vi "Main Editor UI.vi"() -> ()   [LabVIEW 2015, in "Increment editor node.lvclass"]
doc: "This is the main view for configuration the behavior of a module in the DCAF standard editor."
uses:
  Increment editor node.lvclass
  <vilib>/NI/Configuration Framework/Node/NodeRef.ctl
  <vilib>/NI/Configuration Framework/Node/NISE_CEF_Node.lvclass
  <vilib>/NI/AMC/Message Queue.ctl
  <vilib>/NI/AMC/Message.ctl
  <vilib>/NI/Tools/Keyed Array/KeyedArray.ctl
  <vilib>/NI/Configuration Framework/Node/UserEventRef.ctl
  <vilib>/NI/Configuration Framework/Controls/EventCluster.ctl
  <vilib>/NI/DCAF UI Toolkit/Controls/Configure.ctl
  <vilib>/NI/DCAF UI Toolkit/Controls/Add.ctl
  <vilib>/NI/DCAF UI Toolkit/Controls/Remove.ctl
  <vilib>/NI/Configuration Framework/Node/StopEvent.ctl
  <vilib>/NI/Configuration Framework/Node/RefreshUIEvent.ctl
  <vilib>/NI/Configuration Framework/Node/CacheState.ctl
  <vilib>/NI/Configuration Framework/Node/NodeChangeEvent.ctl
  <vilib>/NI/Tag Bus/tag/Data Type.ctl
  Permissions Enum.ctl
  <vilib>/NI/DCAF/Tag Editor Core/Table API/Available Tag Menu/channel action event.ctl
  <vilib>/NI/DCAF/Tag Editor Core/Table API/Available Tag Menu/dialog output action.ctl
  <vilib>/NI/Tag Bus Module Framework/channel/TBM channel.lvclass
  <vilib>/NI/Tag Bus/tag/tag descriptor.lvclass
  <vilib>/NI/DCAF/Tag Editor Core/Table API/Table Manager/Call Back Ref Type Def.ctl
  <vilib>/NI/DCAF/Tag Editor Core/Configuration Editor/Classes/Engine Parent/Engine Parent Editor Node.lvclass
  <vilib>/NI/DCAF/Tag Editor Core/Configuration Editor/Classes/Module editor node/module editor node.lvclass
  <vilib>/NI/DCAF UI Toolkit/Controls/Import.ctl
  <vilib>/NI/DCAF UI Toolkit/Controls/Export.ctl
  <vilib>/NI/DCAF/Tag Editor Core/Table API/Table Manager/references.ctl
  <vilib>/Utility/miscctls.llb/LVPositionTypeDef.ctl
  <vilib>/NI/DCAF/Tag Editor Core/Table API/Listbox/Multi Column Listbox.lvclass
  <vilib>/NI/Configuration Framework/NISE_CEF_TreeControl.lvlib
  <vilib>/NI/Tools/Keyed Array/Tools_KeyedArray.lvlib
  <vilib>/NI/AMC/AMC.lvlib
  <vilib>/NI/DCAF/Tag Editor Core/Table API/Table Manager.lvlib
  <vilib>/NI/DCAF/Tag Editor Core/Table API/Table Manager/Table Manager.lvclass
  <vilib>/NI/DCAF UI Toolkit/Controls/DCAF UI Elements.lvlib
panel:
  in  "user event out":refnum<user-event>
  in  "Permissions":T1
  in  "data type":T2
  in  "node change":T3
  in  "cache state":T4
  in  "refresh UI":T5
  in  "stop event":T6
  in  "Tab Control":enum32{"Channel Configuration", "Import Export"}(tab)
  in  "Remove Button":T7
  in  "Add Button":T8
  in  "Table":i32(listbox)
  in  "settings":T9
  in  "Export":T10
  in  "Import":T11
  in  "user event":T12
  in  "main queue":T13
  in  "node ref":T14
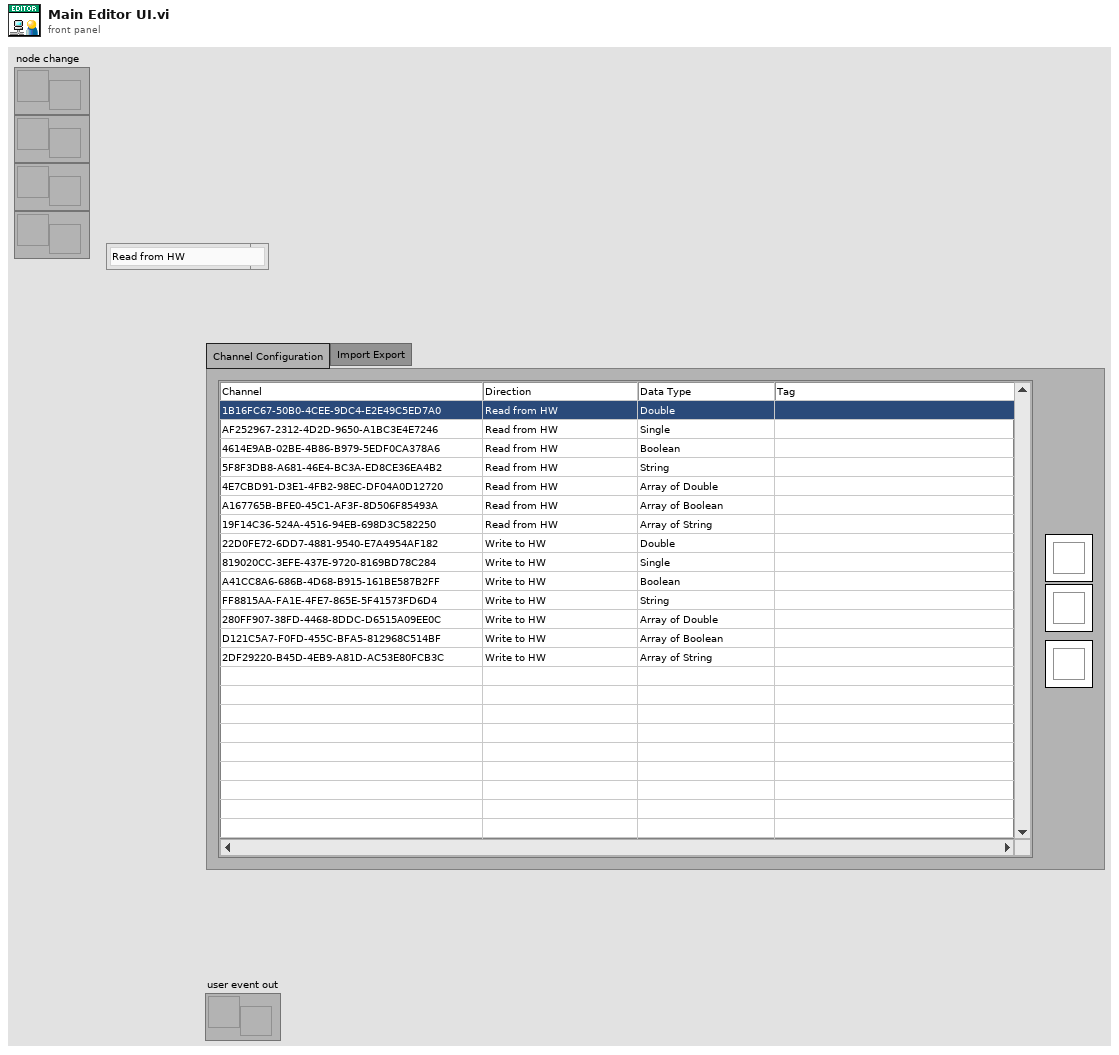
[diagram p1: front panel]
types:
  T1 = typedef "Increment editor node.lvclass/Permissions Enum.ctl" = enum16{"Read from HW", "Write to HW"}
  T2 = typedef "tag bus.lvlib/tag descriptor.lvclass/Data Type.ctl" = enum16{"Double", "Single", "I64", "I32", "I16", "I8", "U64", "U32", "U16", "U8", "Boolean", "String", "Array of Double", "Array of Single", "Array of I64", "Array of I32", "Array of I16", "Array of I8", "Array of U64", "Array of U32", "Array of U16", "Array of U8", "Array of Boolean", "Array of String"}
  T3 = typedef "NISE_CEF_Node.lvclass/NodeChangeEvent.ctl" = refnum<user-event>
  T4 = typedef "NISE_CEF_Node.lvclass/CacheState.ctl" = refnum<user-event>
  T5 = typedef "NISE_CEF_Node.lvclass/RefreshUIEvent.ctl" = refnum<user-event>
  T6 = typedef "NISE_CEF_Node.lvclass/StopEvent.ctl" = refnum<user-event>
  T7 = typedef "DCAF UI Elements.lvlib/Remove.ctl" = bool
  T8 = typedef "DCAF UI Elements.lvlib/Add.ctl" = bool
  T9 = typedef "DCAF UI Elements.lvlib/Configure.ctl" = bool
  T10 = typedef "DCAF UI Elements.lvlib/Export.ctl" = bool
  T11 = typedef "DCAF UI Elements.lvlib/Import.ctl" = bool
  T12 = typedef "NISE_CEF_Node.lvclass/UserEventRef.ctl" = refnum<user-event>
  T13 = typedef "AMC.lvlib/Message Queue.ctl" = refnum<queue>
  T14 = typedef "NISE_CEF_Node.lvclass/NodeRef.ctl" = refnum<data-value>
  T15 = typedef "Table Manager.lvlib/Table Manager.lvclass/references.ctl" = cluster{"stop event":T6, "refresh UI":T5, "cache state":T4, "node change":T3, "user event out":refnum<user-event>, "main queue":T13, "user event":T12}
  T16 = typedef "LVPositionTypeDef.ctl" = cluster{"Left":i32, "Top":i32}
  T17 = typedef "Table Manager.lvlib/Table Manager.lvclass/object ref.ctl" = cluster{"engine":refnum<data-value>, "Node Ref":refnum<data-value>}
  T18 = typedef "Table Manager.lvlib/Column.lvclass/Column Descriptor.ctl" = cluster{"name":string, "caption":string, "Column Type":T19, "Params":string, "AutoSizeMode":i32, "FillWeight":sgl, "MinWidth":u32, "tooltip":string, "Enum Reference":refnum<vi>, "Channel suffix":string, "Read Only":bool, "Call Back VI":T20, "DT Dependency":i32, "name dependency":i32, "data type":T2, "Custom Column":refnum<class "Column.lvclass">}
  T19 = typedef "Table Manager.lvlib/Column.lvclass/Column Type.ctl" = enum16{"String", "Mapping", "Enum", "Custom"}
  T20 = typedef "Table Manager.lvlib/Table Manager.lvclass/Call Back Ref Type Def.ctl" = refnum<vi>
  T21 = typedef "Table Manager.lvlib/Table Manager.lvclass/Table Events.ctl" = cluster{"Menu Selection":refnum<user-event>}
  T22 = enum8{"Enabled", "Disabled", "Disabled and Grayed Out"}
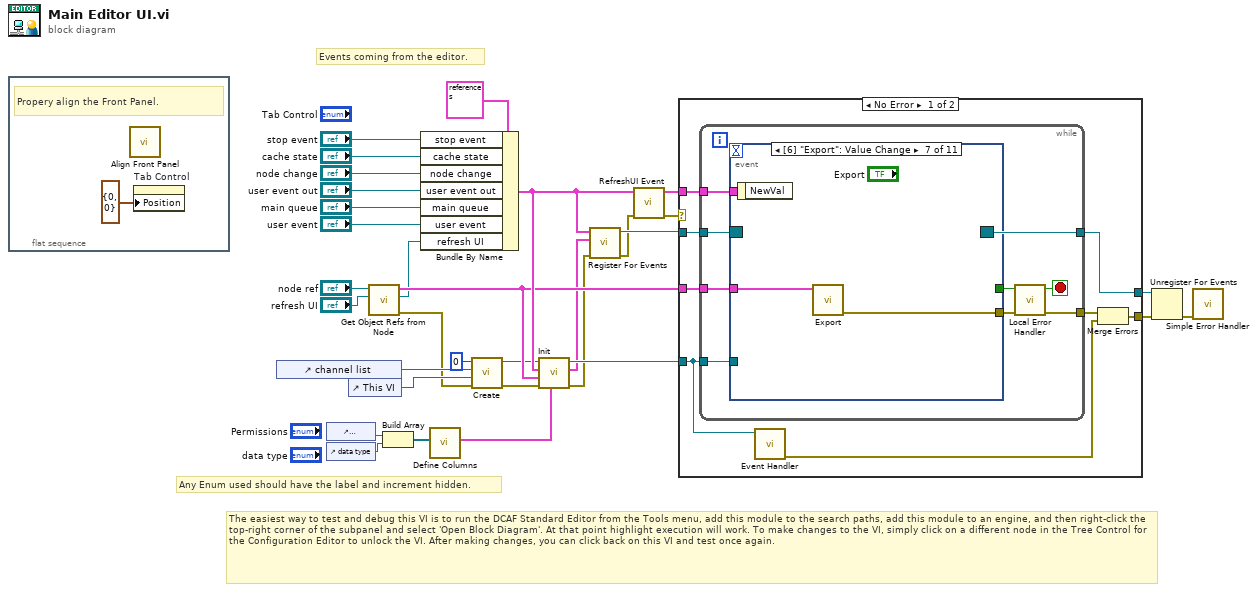
[diagram p0: block diagram]
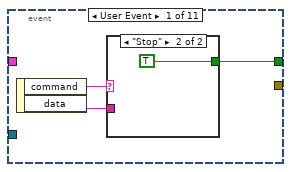
[diagram p2: hidden frame]
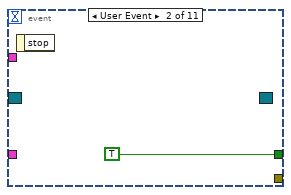
[diagram p4: hidden frame]
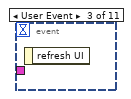
[diagram p5: hidden frame]
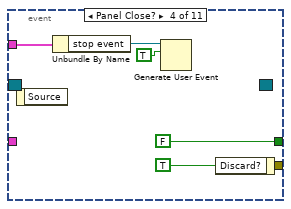
[diagram p6: hidden frame]
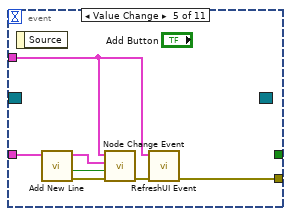
[diagram p7: hidden frame]
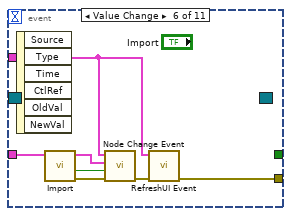
[diagram p8: hidden frame]
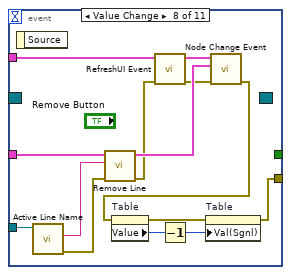
[diagram p9: hidden frame]
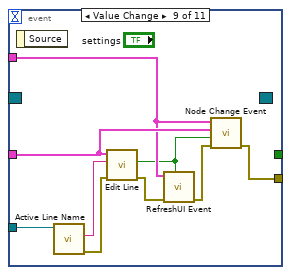
[diagram p10: hidden frame]
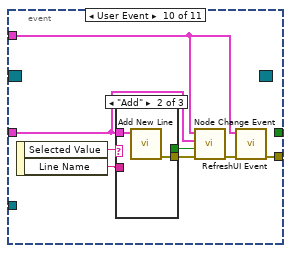
[diagram p11: hidden frame]
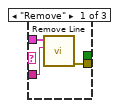
[diagram p12: hidden frame]
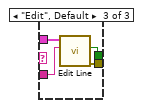
[diagram p13: hidden frame]
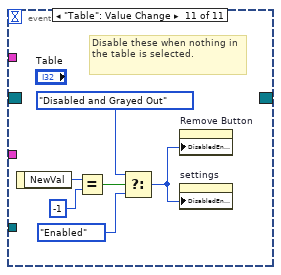
[diagram p14: hidden frame]
diagram:
  # "The easiest way to test and debug this VI is to run the DCAF Standard Editor from the Tools menu, add this module to the search paths, add this module to an engine, and then right-click the top-right corner of the subpanel and select 'Open Block Diagram'. At that point highlight execution will work. To make changes to the VI, simply click on a different node in the Tree Control for the Configuration Editor to unlock the VI. After making changes, you can click back on this VI and test once again."
  # "Any Enum used should have the label and increment hidden."
  # "Events coming from the editor."
  n1 = flat-sequence {
    frame #0 {
      # "Propery align the Front Panel."
      n2 = call <vilib>:"Align Front Panel.vi"() -> ()  [unwired: 10 in, 2 out]
      n3 = property on="Tab Control" class="TabCtl (strict)"("Position"=T16 {"Left"=0, "Top"=0}) -> ()  [unwired: 2 in, 2 out]
    }
  }
  n4 = control-ref of="channel list"() -> (w8:refnum<vi>)
  n5 = control-ref of="Permissions"() -> (w18:refnum<vi>)
  n6 = control-ref of="data type"() -> (w17:refnum<vi>)
  n7 = control-ref of="This VI"() -> (w6:refnum<vi>)
  n8 = call "Get Object Refs from Node.vi"("Refresh UI"="refresh UI", "Data Value Reference in"="node ref") -> ("error out"=w3:errorcluster, "Refresh UI out"=w1:T5, "References"=w15:T17)  [unwired: 7 in]
  n9 = Build Array(w18, w17) -> (w16:refnum<vi>[])
  n10 = Bundle By Name(cluster=T15 {"stop event"=refnum, "refresh UI"=refnum, "cache state"=refnum, "node change"=refnum, "user event out"=refnum, "main queue"=refnum, "user event"=refnum} ("References"), "stop event"="stop event", "cache state"="cache state", "node change"="node change", "user event out"="user event out", "main queue"="main queue", "user event"="user event", "refresh UI"=w1) -> (w19:T15)
  n11 = call "Define Columns.vi"("Enum Array"=w16) -> ("Column Definition"=w21:T18[])  [unwired: 10 in]
  n12 = call <vilib>:"Create.vi"("error in (no error)"=w3, "Top VI"=w6, "Listbox"=w8, "Index"=0) -> ("error out"=w4:errorcluster, "reference out"=w5:refnum<class "Multi Column Listbox.lvclass">)  [unwired: 6 in]
  n13 = call-dynamic "Init.vi"("Column Descriptors"=w21, "error in (no error)"=w4, "Node object refs"=w15, "Event References"=w19, "Multi Column Listbox in"=w5) -> ("error out"=w10:errorcluster, "Table Events"=w9:T21, "Multi Column Listbox out"=w14:refnum<class "Multi Column Listbox.lvclass">)  [unwired: 4 in]
  n14 = call "Register For Events.vi"("error in"=w10, "Table Events"=w9, "References"=w19) -> ("error out"=w12:errorcluster, "Event Registration Refnum"=w22:refnum<event-registration>)  [unwired: 7 in]
  n15 = call "RefreshUI Event.vi"("error in (no error)"=w12, "References in"=w19) -> ("error out"=w11:errorcluster, "References out"=w20:T15)  [unwired: 8 in]
  n16 = case shown="No Error" w11 {
    selector: w11 -> [_ w122]
    tunnel: w22 -> [w41 w121]
    tunnel: [w40 w121] -> w32
    tunnel: [w34 w122] -> w31
    tunnel: w20 -> [w39 _]
    tunnel: w15 -> [w38 _]
    tunnel: w14 -> [w37 _]
    frame No Error {
      n17 = while {
        tunnel: w41 -> [w50]
        tunnel: [w49] -> w40
        tunnel: [w46] -> w35
        tunnel: w39 -> [w44]
        tunnel: w38 -> [w43]
        tunnel: w37 -> [w42]
        stop <- w48 stop-if-true
        n18 = event shown="[6] \"Export\": Value Change" {
          selector: w50 -> [_ _ _ _ _ _ _ _ _ _ _]
          dyn-events: [_ _ _ _ _ _ _ _ _ _ _] -> w49
          timeout: _ -> [_ _ _ _ _ _ _ _ _ _ _]
          tunnel: [w53 TRUE _ FALSE _ _ _ _ _ _ _] -> w47
          tunnel: [_ _ _ _ w61 w71 w74 w77 w97 w103 _] -> w45
          tunnel: w44 -> [_ _ _ w57 w65 w73 _ w88 w92 w99 _]
          tunnel: w43 -> [_ _ _ _ w66 w70 w75 w87 w95 w100 _]
          tunnel: w42 -> [_ _ _ _ _ _ _ w83 w96 _ _]
          event User Event {
            n19 = event-data() -> ("command"=w52:string, "data"=w51:string)  [unwired: 1 in]
            n20 = case shown="\"Stop\"" w52 {
              tunnel: [_ TRUE] -> w53
              tunnel: w51 -> [_ _]
              frame Default {
              }
              frame "Stop" {
              }
            }
          }
          event User Event {
            n21 = event-data() -> ()  [unwired: 1 in, 1 out]
          }
          event User Event {
            n22 = event-data() -> ()  [unwired: 1 in, 1 out]
          }
          event Panel Close? {
            n23 = event-data() -> ()  [unwired: 1 in, 1 out]
            n24 = Unbundle By Name(w57) -> ("stop event"=w56:T6)
            n25 = Generate User Event(user event=w56, event data cluster=TRUE ("event data")) -> ()  [unwired: 2 in, 2 out]
            n26 = event-data("Discard?"=TRUE) -> ()  [unwired: 1 in, 1 out]
          }
          event Value Change {
            n27 = event-data() -> ()  [unwired: 1 in, 1 out]
            n28 = call "Add New Line.vi"("objects"=w66) -> ("error out"=w64:errorcluster, "success"=w62:bool)  [unwired: 8 in, 1 out]
            n29 = call "Node Change Event.vi"("error in (no error)"=w64, "Send (T)"=w62, "objects"=w66, "References in"=w65) -> ("error out"=w63:errorcluster)  [unwired: 7 in]
            n30 = call "RefreshUI Event.vi"("error in (no error)"=w63, "References in"=w65) -> ("error out"=w61:errorcluster)  [unwired: 8 in, 1 out]
          }
          event Value Change {
            n31 = event-data() -> ()  [unwired: 1 in, 6 out]
            n32 = call "Import.vi"("Objects in"=w70) -> ("error out"=w67:errorcluster, "Update"=w68:bool, "Objects out"=w69:T17)  [unwired: 8 in]
            n33 = call "Node Change Event.vi"("error in (no error)"=w67, "Send (T)"=w68, "objects"=w69, "References in"=w73) -> ("error out"=w72:errorcluster)  [unwired: 7 in]
            n34 = call "RefreshUI Event.vi"("error in (no error)"=w72, "References in"=w73) -> ("error out"=w71:errorcluster)  [unwired: 8 in, 1 out]
          }
          event Value Change {
            n35 = event-data() -> ()  [unwired: 1 in, 1 out]
            n36 = call "Export.vi"("Objects"=w75) -> ("error out"=w74:errorcluster)  [unwired: 10 in]
          }
          event Value Change {
            n37 = event-data() -> ()  [unwired: 1 in, 1 out]
            n38 = call-dynamic "Active Line Name.vi"("Multi Column Listbox in"=w83) -> ("error out"=w81:errorcluster, "Active Line Name"=w82:string)  [unwired: 8 in, 1 out]
            n39 = call "Remove Line.vi"("error in"=w81, "Active Line Name"=w82, "Objects"=w87) -> ("error out"=w84:errorcluster)  [unwired: 8 in]
            n40 = call "RefreshUI Event.vi"("error in (no error)"=w84, "References in"=w88) -> ("error out"=w86:errorcluster, "References out"=w85:T15)  [unwired: 8 in]
            n41 = call "Node Change Event.vi"("error in (no error)"=w86, "objects"=w87, "References in"=w85) -> ("error out"=w78:errorcluster)  [unwired: 8 in]
            n42 = property on="Table" class="MCListbox (strict)"(error in=w78) -> (error out=w76:errorcluster, "Value"=w79:i32)  [unwired: 1 in, 1 out]
            n43 = Decrement(x=w79) -> (x-1=w80:i32)
            n44 = property on="Table" class="MCListbox (strict)"(error in=w76, "Val(Sgnl)"=w80) -> (error out=w77:errorcluster)  [unwired: 1 in, 1 out]
          }
          event Value Change {
            n45 = event-data() -> ()  [unwired: 1 in, 1 out]
            n46 = call-dynamic "Active Line Name.vi"("Multi Column Listbox in"=w96) -> ("error out"=w93:errorcluster, "Active Line Name"=w94:string)  [unwired: 8 in, 1 out]
            n47 = call "Edit Line.vi"("error in"=w93, "Line Name"=w94, "References"=w95) -> ("error out"=w90:errorcluster, "change?"=w91:bool)  [unwired: 7 in]
            n48 = call "RefreshUI Event.vi"("Refresh (T)"=w91, "error in (no error)"=w90, "References in"=w92) -> ("error out"=w89:errorcluster)  [unwired: 7 in, 1 out]
            n49 = call "Node Change Event.vi"("error in (no error)"=w89, "Send (T)"=w91, "objects"=w95, "References in"=w92) -> ("error out"=w97:errorcluster)  [unwired: 7 in]
          }
          event User Event {
            n50 = event-data() -> ("Selected Value"=w105:string, "Line Name"=w102:string)  [unwired: 1 in]
            n51 = case shown="\"Add\"" w105 {
              tunnel: w102 -> [w108 _ w114]
              tunnel: w100 -> [w107 w110 w113]
              tunnel: [w106 w109 w112] -> w101
              tunnel: [_ _ w111] -> w98
              frame "Remove" {
                n52 = call "Remove Line.vi"("Active Line Name"=w108, "Objects"=w107) -> ("error out"=w106:errorcluster)  [unwired: 9 in]
              }
              frame "Add" {
                n53 = call "Add New Line.vi"("objects"=w110) -> ("error out"=w109:errorcluster)  [unwired: 8 in, 2 out]
              }
              frame "Edit", Default {
                n54 = call "Edit Line.vi"("Line Name"=w114, "References"=w113) -> ("error out"=w112:errorcluster, "change?"=w111:bool)  [unwired: 8 in]
              }
            }
            n55 = call "Node Change Event.vi"("error in (no error)"=w101, "Send (T)"=w98, "objects"=w100, "References in"=w99) -> ("error out"=w104:errorcluster)  [unwired: 7 in]
            n56 = call "RefreshUI Event.vi"("error in (no error)"=w104, "References in"=w99) -> ("error out"=w103:errorcluster)  [unwired: 8 in, 1 out]
          }
          event "Table": Value Change {
            # "Disable these when nothing in the table is selected."
            n57 = event-data() -> ("NewVal"=w120:i32)  [unwired: 1 in]
            n58 = Equal?(x=w120, y=-1) -> (x = y?=w118:bool)
            n59 = Select(t=T22."Disabled and Grayed Out" ("Disabled"), s=w118, f=T22."Enabled") -> (s? t:f=w116:T22)
            n60 = property on="Remove Button" class="Bool"("DisabledEnum"=w116) -> ()  [unwired: 2 in, 2 out]
            n61 = property on="settings" class="Bool"("DisabledEnum"=w116) -> ()  [unwired: 2 in, 2 out]
          }
        }
        n62 = call "Local Error Handler.vi"("error in"=w45, "Stop in"=w47) -> ("error out"=w46:errorcluster, "Stop out"=w48:bool)  [unwired: 8 in]
      }
      n63 = call-dynamic "Event Handler.vi"("Listbox in"=w37) -> ("error out"=w36:errorcluster)  [unwired: 9 in, 1 out]
      n64 = Merge Errors(w35, w36) -> (w34:errorcluster)
    }
    frame Error {
    }
  }
  n65 = Unregister For Events(event registration refnum=w32, error in=w31) -> (error out=w30:errorcluster)
  n66 = call <vilib>:"Simple Error Handler.vi"("error in (no error)"=w30) -> ()  [unwired: 4 in, 5 out]
